vi "Add.vi"(10 "Element":variant=variant(i32 0), 11 "TypedCircularBuffer in":refnum<class "VarCircularBuffer.lvclass">) -> (1 "overflow?":bool, 2 "overflow element":variant=variant(i32 0), 3 "TypedCircularBuffer out":refnum<class "VarCircularBuffer.lvclass">)   [LabVIEW 2024, in "VarCircularBuffer.lvclass"]
uses:
  VarCircularBuffer.lvclass
  VarCircularBuffer.lvclass/VarCircularBuffer.ctl
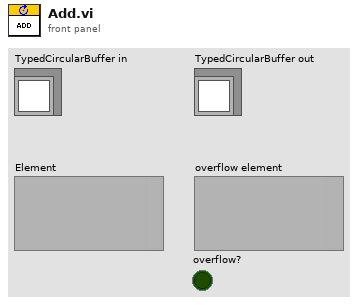
[diagram p1: front panel]
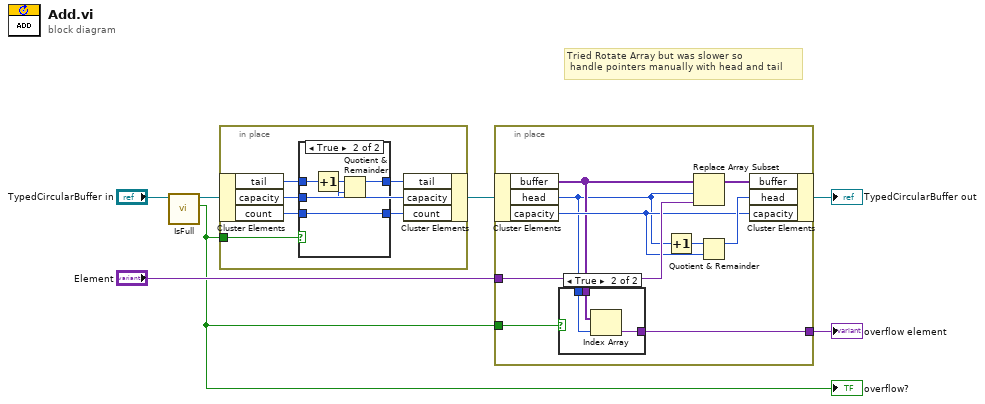
[diagram p0: block diagram]
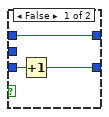
[diagram p2: hidden frame]
diagram:
  # "Tried Rotate Array but was slower so\n handle pointers manually with head and tail"
  n1 = call "IsFull.vi"("TypedCircularBuffer in"="TypedCircularBuffer in") -> ("Full?"=w1:bool, "TypedCircularBuffer out"=w3:refnum<class "VarCircularBuffer.lvclass">)  [unwired: 9 in]
  "overflow?" <- w1
  n2 = in-place {
    in-place-border: w1 -> [w8]
    n3 = in-place-cluster #1(w3) -> ("tail"=w13:u32, "capacity"=w10:u32, "count"=w9:u32)
    n4 = case shown="True" w8 {
      tunnel: w13 -> [w16 w20]
      tunnel: w10 -> [_ w19]
      tunnel: [w16 w18] -> w12
      tunnel: w9 -> [w15 w17]
      tunnel: [w14 w17] -> w11
      frame False {
        n5 = Increment(x=w15) -> (x+1=w14:u32)
      }
      frame True {
        n6 = Increment(x=w20) -> (x+1=w21:u32)
        n7 = Quotient & Remainder(x=w21, y=w19) -> (x-y*floor(x/y)=w18:u32)  [unwired: 1 out]
      }
    }
    n8 = in-place-cluster #1("tail"=w12, "capacity"=w10, "count"=w11) -> (w4:refnum<class "VarCircularBuffer.lvclass">)
  }
  n9 = in-place {
    in-place-border: "Element" -> [w29]
    in-place-border: [w24] -> w2
    in-place-border: w1 -> [w22]
    n10 = in-place-cluster #2(w4) -> ("buffer"=w25:variant[], "head"=w23:u32, "capacity"=w27:u32)
    n11 = case shown="True" w22 {
      tunnel: w25 -> [_ w33]
      tunnel: [_ w32] -> w24
      tunnel: w23 -> [_ w31]
      frame False {
      }
      frame True {
        n12 = Index Array(array=w33, index=w31) -> (element=w32:variant)
      }
    }
    n13 = Increment(x=w23) -> (x+1=w26:u32)
    n14 = Replace Array Subset(array=w25, new element=w29, index=w23) -> (w28:variant[])
    n15 = Quotient & Remainder(x=w26, y=w27) -> (x-y*floor(x/y)=w30:u32)  [unwired: 1 out]
    n16 = in-place-cluster #2("buffer"=w28, "head"=w30, "capacity"=w27) -> (→"TypedCircularBuffer out":refnum<class "VarCircularBuffer.lvclass">)
  }
  "overflow element" <- w2
